vi "update.vi"(8 "error in (no error)":errorcluster, 10 "Model in":refnum<class "Model.lvclass">, 11 "DisabledState in":refnum<class "DisabledState.lvclass">) -> (0 "error out":errorcluster, 2 "Model out":refnum<class "Model.lvclass">, 3 "DisabledState out":refnum<class "DisabledState.lvclass">)   [LabVIEW 2016, in "DisabledState.lvclass"]
uses:
  DisabledState.lvclass
  Model/Model.lvclass
  Model/Model.lvclass/Model.ctl
  ILCCommunications/ILCCommunications.lvclass/ILCCommunications.ctl
  Common_RT_HPILC/HPILC/HPILC.lvclass/HPILC.ctl
  Common_RT_ILC/ILC/ILC.lvclass/ILC.ctl
  Common_RT_Modbus/ModbusBuffer/ModbusBuffer.lvclass/ModbusBuffer.ctl
  Common_RT_FAILC/FAILC/FAILC.lvclass/FAILC.ctl
  Publisher/Publisher.lvclass/Publisher.ctl
  Communicator/M1M3SAL/M1M3SAL.lvclass/M1M3SAL.ctl
  ILCCommunications/broadcastHPFreezeSensorValues.vi
  ILCCommunications/broadcastFAFreezeSensorValues.vi
  ILCCommunications/reportAllHPForceAndStatus.vi
  ILCCommunications/reportAllFAForceAndStatus.vi
  ILCCommunications/reportAllHPServerStatus.vi
  Model/getFPGA.vi
  Model/setFPGA.vi
  ILCCommunications/parse.vi
  Publisher/transmit.vi
  Common_RT_HPILC/HPILC/addBroadcastFreezeSensorValuesFrame.vi
  Common_RT_FAILC/FAILC/addBroadcastFreezeSensorValuesFrame.vi
  ILCCommunications/reportHPForceAndStatus.vi
  ILCCommunications/reportFAForceAndStatus.vi
  ILCCommunications/reportHPServerStatus.vi
  Common_RT_Modbus/ModbusBuffer/endOfBuffer.vi
  Common_RT_Modbus/ModbusBuffer/readHeader.vi
  Common_RT_Modbus/ModbusBuffer/readU8.vi
  ILCCommunications/findILCMap.vi
  ILCCommunications/getHPs.vi
  ILCCommunications/setHPs.vi
  Common_RT_HPILC/HPILC/parseHP.vi
  ILCCommunications/getFAs.vi
  ILCCommunications/setFAs.vi
  Common_RT_FAILC/FAILC/parseFA.vi
  Communicator/M1M3SAL/transmit.vi
  Common_RT_Modbus/ModbusBuffer/writeHeader.vi
  Common_RT_Modbus/ModbusBuffer/writeU8.vi
  Common_RT_Modbus/ModbusBuffer/writeCRC.vi
  Common_RT_Modbus/ModbusBuffer/writeDelay.vi
  Common_RT_ILC/ILC/getILCData.vi
  Common_RT_Modbus/ModbusBuffer/writeEndOfFrame.vi
  Common_RT_HPILC/HPILC/createForceAndStatusFrame.vi
  Common_RT_FAILC/FAILC/addForceAndStatusFrame.vi
  ILCCommunications/reportServerStatus.vi
  Common_RT_Modbus/ModbusBuffer/readInstructionByte.vi
  ILCCommunications/getILCMap.vi
  Common_RT_ILC/ILC/parseILC.vi
  Common_RT_HPILC/HPILC/parseStepMotorResponse.vi
  Common_RT_HPILC/HPILC/parseStepMotorError.vi
  Common_RT_HPILC/HPILC/parseForceAndStatusResponse.vi
  Common_RT_HPILC/HPILC/parseForceAndStatusError.vi
  Common_RT_FAILC/FAILC/parseBoosterValveGainResponse.vi
  Common_RT_FAILC/FAILC/parseBoosterValveGainError.vi
  Common_RT_FAILC/FAILC/parseReadBoosterValveGainResponse.vi
  Common_RT_FAILC/FAILC/parseReadBoosterValveGainError.vi
  Common_RT_FAILC/FAILC/parseSetForceResponse.vi
  Common_RT_FAILC/FAILC/parseSetForceError.vi
  Common_RT_FAILC/FAILC/parseForceAndStatusResponse.vi
  Common_RT_FAILC/FAILC/parseForceAndStatusError.vi
  Communicator/M1M3SAL/write.vi
  Common_RT_Modbus/ModbusBuffer/writeByteInstruction.vi
  Common_RT_Modbus/ModbusBuffer/calculateCRC.vi
  Common_RT_Modbus/ModbusBuffer/writeWaitForRx.vi
  Common_RT_ILC/ILC/addReportServerStatusFrame.vi
  Common_RT_ILC/ILC/parseReportServerIDFrame.vi
  Common_RT_ILC/ILC/parseReportServerIDError.vi
  Common_RT_ILC/ILC/parseReportServerStatusFrame.vi
  Common_RT_ILC/ILC/parseReportServerStatusError.vi
  Common_RT_ILC/ILC/parseModeFrame.vi
  Common_RT_ILC/ILC/parseModeError.vi
  Common_RT_ILC/ILC/parseTemporaryAddressFrame.vi
  Common_RT_ILC/ILC/parseTemporaryAddressError.vi
  Common_RT_ILC/ILC/parseADCScanRateFrame.vi
  Common_RT_ILC/ILC/parseADCScanRateError.vi
  Common_RT_ILC/ILC/parseADCOffsetSensitivityFrame.vi
  Common_RT_ILC/ILC/parseADCOffsetSensitivityError.vi
  Common_RT_ILC/ILC/parseResetFrame.vi
  Common_RT_ILC/ILC/parseResetError.vi
  Common_RT_ILC/ILC/parseReportCalibrationDataFrame.vi
  Common_RT_ILC/ILC/parseReportCalibrationDataError.vi
  Common_RT_Modbus/ModbusBuffer/readCRC.vi
  Common_RT_Modbus/ModbusBuffer/readTimestamp.vi
  Common_RT_Modbus/ModbusBuffer/readEndOfFrame.vi
  Common_RT_Modbus/ModbusBuffer/readI32.vi
  Common_RT_Modbus/ModbusBuffer/readSGL.vi
  Common_RT_Modbus/ModbusBuffer/readU48.vi
  Common_RT_Modbus/ModbusBuffer/readString.vi
  Common_RT_Modbus/ModbusBuffer/readU16.vi
  Common_RT_Modbus/ModbusBuffer/readTimestampByte.vi
  Common_RT_HPILC/HPILC/HPILC.lvclass
  D:/Code/ts_M1M3Support/Common_RT_ILC/ILC/ILC.lvclass
  Common_RT_FAILC/FAILC/FAILC.lvclass
  Resources/FPGA/writeModbusTxData.vi
  Resources/FPGA/writeModbusTrigger.vi
  Resources/FPGA/writeHealthAndStatusControl.vi
  Resources/FPGA/readModbusRxData.vi
panel:
  out "Total Time (us)":u32
  out "Times (us)":u32[](array[numeric])
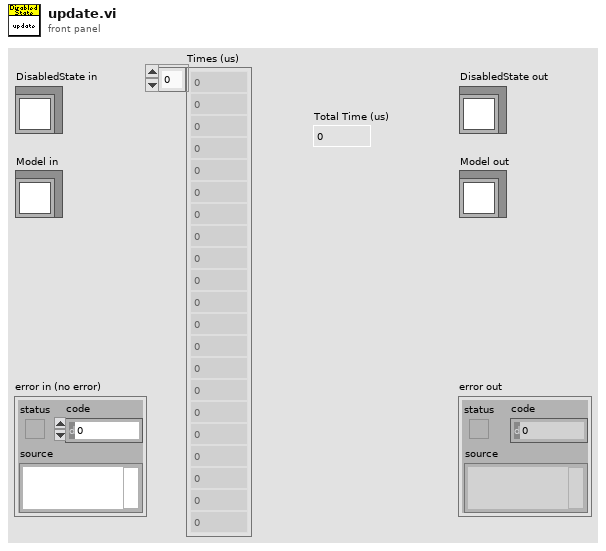
[diagram p1: front panel]
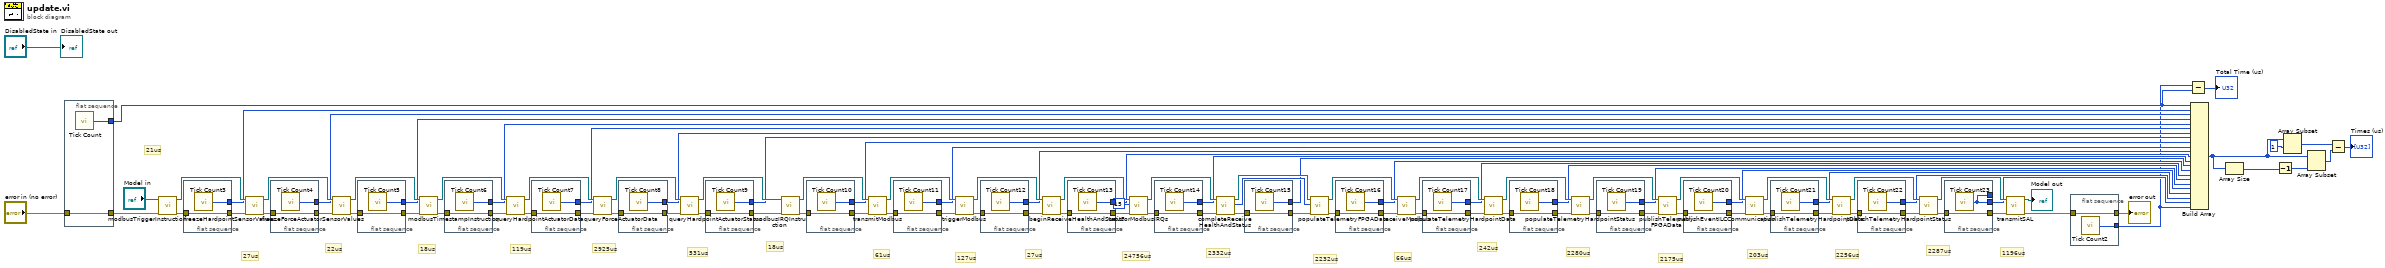
[diagram p0: block diagram]
diagram:
  # "1196us"
  # "2287us"
  # "2256us"
  # "203us"
  # "2175us"
  # "2280us"
  # "242us"
  # "66us"
  # "2232us"
  # "2332us"
  # "24756us"
  # "27us"
  # "127us"
  # "61us"
  # "531us"
  # "2925us"
  # "119us"
  # "18us"
  # "22us"
  # "27us"
  # "21us"
  # "18us"
  n1 = flat-sequence {
    tunnel: "error in (no error)" -> [w104]
    tunnel: [w105] -> w4
    tunnel: [w104] -> w79
    frame #0 {
      n2 = call "Tick Count"() -> ("Tick Count(uSec)"=w105:u32)
    }
  }
  n3 = call "modbusTriggerInstruction.vi"("error in (no error)"=w79, "Model in"="Model in") -> ("error out"=w75:errorcluster, "Model out"=w90:refnum<class "Model.lvclass">)  [unwired: 8 in]
  n4 = flat-sequence {
    tunnel: w75 -> [w107]
    tunnel: [w106] -> w67
    tunnel: [w107] -> w74
    frame #0 {
      n5 = call "Tick Count3"() -> ("Tick Count(uSec)"=w106:u32)
    }
  }
  n6 = call "freezeHardpointSensorValues.vi"("error in (no error)"=w74, "Model in"=w90) -> ("error out"=w73:errorcluster, "Model out"=w84:refnum<class "Model.lvclass">)  [unwired: 8 in]
  n7 = flat-sequence {
    tunnel: w73 -> [w109]
    tunnel: [w108] -> w66
    tunnel: [w109] -> w72
    frame #0 {
      n8 = call "Tick Count4"() -> ("Tick Count(uSec)"=w108:u32)
    }
  }
  n9 = call "freezeForceActuatorSensorValues.vi"("error in (no error)"=w72, "Model in"=w84) -> ("error out"=w71:errorcluster, "Model out"=w83:refnum<class "Model.lvclass">)  [unwired: 8 in]
  n10 = flat-sequence {
    tunnel: w71 -> [w111]
    tunnel: [w110] -> w65
    tunnel: [w111] -> w70
    frame #0 {
      n11 = call "Tick Count5"() -> ("Tick Count(uSec)"=w110:u32)
    }
  }
  n12 = call "modbusTimestampInstruction.vi"("error in (no error)"=w70, "Model in"=w83) -> ("error out"=w69:errorcluster, "Model out"=w91:refnum<class "Model.lvclass">)  [unwired: 8 in]
  n13 = flat-sequence {
    tunnel: w69 -> [w113]
    tunnel: [w112] -> w64
    tunnel: [w113] -> w68
    frame #0 {
      n14 = call "Tick Count6"() -> ("Tick Count(uSec)"=w112:u32)
    }
  }
  n15 = call "queryHardpointActuatorData.vi"("error in (no error)"=w68, "Model in"=w91) -> ("error out"=w63:errorcluster, "Model out"=w82:refnum<class "Model.lvclass">)  [unwired: 8 in]
  n16 = flat-sequence {
    tunnel: w63 -> [w115]
    tunnel: [w114] -> w57
    tunnel: [w115] -> w62
    frame #0 {
      n17 = call "Tick Count7"() -> ("Tick Count(uSec)"=w114:u32)
    }
  }
  n18 = call "queryForceActuatorData.vi"("error in (no error)"=w62, "Model in"=w82) -> ("error out"=w61:errorcluster, "Model out"=w81:refnum<class "Model.lvclass">)  [unwired: 8 in]
  n19 = flat-sequence {
    tunnel: w61 -> [w117]
    tunnel: [w116] -> w56
    tunnel: [w117] -> w60
    frame #0 {
      n20 = call "Tick Count8"() -> ("Tick Count(uSec)"=w116:u32)
    }
  }
  n21 = call "queryHardpointActuatorStatus.vi"("error in (no error)"=w60, "Model in"=w81) -> ("error out"=w59:errorcluster, "Model out"=w94:refnum<class "Model.lvclass">)  [unwired: 8 in]
  n22 = flat-sequence {
    tunnel: w59 -> [w119]
    tunnel: [w118] -> w55
    tunnel: [w119] -> w58
    frame #0 {
      n23 = call "Tick Count9"() -> ("Tick Count(uSec)"=w118:u32)
    }
  }
  n24 = call "modbusIRQInstruction.vi"("error in (no error)"=w58, "Model in"=w94) -> ("error out"=w54:errorcluster, "Model out"=w93:refnum<class "Model.lvclass">)  [unwired: 8 in]
  n25 = flat-sequence {
    tunnel: w54 -> [w121]
    tunnel: [w120] -> w40
    tunnel: [w121] -> w53
    frame #0 {
      n26 = call "Tick Count10"() -> ("Tick Count(uSec)"=w120:u32)
    }
  }
  n27 = call "transmitModbus.vi"("error in (no error)"=w53, "Model in"=w93) -> ("error out"=w52:errorcluster, "Model out"=w92:refnum<class "Model.lvclass">)  [unwired: 8 in]
  n28 = flat-sequence {
    tunnel: w52 -> [w123]
    tunnel: [w122] -> w39
    tunnel: [w123] -> w51
    frame #0 {
      n29 = call "Tick Count11"() -> ("Tick Count(uSec)"=w122:u32)
    }
  }
  n30 = call "triggerModbus.vi"("error in (no error)"=w51, "Model in"=w92) -> ("error out"=w50:errorcluster, "Model out"=w89:refnum<class "Model.lvclass">)  [unwired: 8 in]
  n31 = flat-sequence {
    tunnel: w50 -> [w125]
    tunnel: [w124] -> w38
    tunnel: [w125] -> w49
    frame #0 {
      n32 = call "Tick Count12"() -> ("Tick Count(uSec)"=w124:u32)
    }
  }
  n33 = call "beginReceiveHealthAndStatus.vi"("error in (no error)"=w49, "Model in"=w89) -> ("error out"=w48:errorcluster, "Model out"=w102:refnum<class "Model.lvclass">)  [unwired: 8 in]
  n34 = flat-sequence {
    tunnel: w48 -> [w127]
    tunnel: [w126] -> w37
    tunnel: [w127] -> w47
    frame #0 {
      n35 = call "Tick Count13"() -> ("Tick Count(uSec)"=w126:u32)
    }
  }
  n36 = call "waitForModbusIRQs.vi"("error in (no error)"=w47, "Timeout (ms)"=15, "Model in"=w102) -> ("error out"=w46:errorcluster, "Model out"=w88:refnum<class "Model.lvclass">)  [unwired: 7 in]
  n37 = flat-sequence {
    tunnel: w46 -> [w129]
    tunnel: [w128] -> w36
    tunnel: [w129] -> w45
    frame #0 {
      n38 = call "Tick Count14"() -> ("Tick Count(uSec)"=w128:u32)
    }
  }
  n39 = call "completeReceiveHealthAndStatus.vi"("error in (no error)"=w45, "Model in"=w88) -> ("error out"=w44:errorcluster, "Data"=w101:u64[], "Model out"=w100:refnum<class "Model.lvclass">)  [unwired: 7 in]
  n40 = flat-sequence {
    tunnel: w44 -> [w131]
    tunnel: [w130] -> w35
    tunnel: [w131] -> w43
    frame #0 {
      n41 = call "Tick Count15"() -> ("Tick Count(uSec)"=w130:u32)
    }
  }
  n42 = call "populateTelemetryFPGAData.vi"("error in (no error)"=w43, "Data"=w101, "Model in"=w100) -> ("error out"=w42:errorcluster, "Model out"=w87:refnum<class "Model.lvclass">)  [unwired: 7 in]
  n43 = flat-sequence {
    tunnel: w42 -> [w133]
    tunnel: [w132] -> w34
    tunnel: [w133] -> w41
    frame #0 {
      n44 = call "Tick Count16"() -> ("Tick Count(uSec)"=w132:u32)
    }
  }
  n45 = call "receiveModbus.vi"("error in (no error)"=w41, "Model in"=w87) -> ("error out"=w33:errorcluster, "Model out"=w86:refnum<class "Model.lvclass">)  [unwired: 8 in]
  n46 = flat-sequence {
    tunnel: w33 -> [w135]
    tunnel: [w134] -> w18
    tunnel: [w135] -> w32
    frame #0 {
      n47 = call "Tick Count17"() -> ("Tick Count(uSec)"=w134:u32)
    }
  }
  n48 = call "populateTelemetryHardpointData.vi"("error in (no error)"=w32, "Model in"=w86) -> ("error out"=w31:errorcluster, "Model out"=w99:refnum<class "Model.lvclass">)  [unwired: 8 in]
  n49 = flat-sequence {
    tunnel: w31 -> [w137]
    tunnel: [w136] -> w17
    tunnel: [w137] -> w30
    frame #0 {
      n50 = call "Tick Count18"() -> ("Tick Count(uSec)"=w136:u32)
    }
  }
  n51 = call "populateTelemetryHardpointStatus.vi"("error in (no error)"=w30, "Model in"=w99) -> ("error out"=w29:errorcluster, "Model out"=w97:refnum<class "Model.lvclass">)  [unwired: 8 in]
  n52 = flat-sequence {
    tunnel: w29 -> [w139]
    tunnel: [w138] -> w16
    tunnel: [w139] -> w28
    frame #0 {
      n53 = call "Tick Count19"() -> ("Tick Count(uSec)"=w138:u32)
    }
  }
  n54 = call "publishTelemetryFPGAData.vi"("error in (no error)"=w28, "Model in"=w97) -> ("error out"=w27:errorcluster, "Model out"=w96:refnum<class "Model.lvclass">)  [unwired: 8 in]
  n55 = flat-sequence {
    tunnel: w27 -> [w141]
    tunnel: [w140] -> w15
    tunnel: [w141] -> w26
    frame #0 {
      n56 = call "Tick Count20"() -> ("Tick Count(uSec)"=w140:u32)
    }
  }
  n57 = call "publishEventILCCommunication.vi"("error in (no error)"=w26, "Model in"=w96) -> ("error out"=w25:errorcluster, "Model out"=w95:refnum<class "Model.lvclass">)  [unwired: 8 in]
  n58 = flat-sequence {
    tunnel: w25 -> [w143]
    tunnel: [w142] -> w14
    tunnel: [w143] -> w24
    frame #0 {
      n59 = call "Tick Count21"() -> ("Tick Count(uSec)"=w142:u32)
    }
  }
  n60 = call "publishTelemetryHardpointData.vi"("error in (no error)"=w24, "Model in"=w95) -> ("error out"=w23:errorcluster, "Model out"=w98:refnum<class "Model.lvclass">)  [unwired: 8 in]
  n61 = flat-sequence {
    tunnel: w23 -> [w145]
    tunnel: [w144] -> w13
    tunnel: [w145] -> w22
    frame #0 {
      n62 = call "Tick Count22"() -> ("Tick Count(uSec)"=w144:u32)
    }
  }
  n63 = call "publishTelemetryHardpointStatus.vi"("error in (no error)"=w22, "Model in"=w98) -> ("error out"=w21:errorcluster, "Model out"=w77:refnum<class "Model.lvclass">)  [unwired: 8 in]
  n64 = flat-sequence {
    tunnel: w21 -> [w147]
    tunnel: [w146] -> _
    tunnel: [w147] -> w20
    tunnel: [w146] -> w12
    frame #0 {
      n65 = call "Tick Count23"() -> ("Tick Count(uSec)"=w146:u32)
    }
  }
  n66 = call "transmitSAL.vi"("error in (no error)"=w20, "Model in"=w77) -> ("error out"=w78:errorcluster, "Model out"=→"Model out":refnum<class "Model.lvclass">)  [unwired: 8 in]
  n67 = flat-sequence {
    tunnel: w78 -> [w148]
    tunnel: [w149] -> w3
    tunnel: [w148] -> w19
    frame #0 {
      n68 = call "Tick Count2"() -> ("Tick Count(uSec)"=w149:u32)
    }
  }
  n69 = Subtract(x=w3, y=w4) -> (x-y=→"Total Time (us)":u32)
  n70 = Build Array(w4, w67, w66, w65, w64, w57, w56, w55, w40, w39, w38, w37, w36, w35, w34, w18, w17, w16, w15, w14, w13, w12, w3) -> (w11:u32[])
  n71 = Array Size(array=w11) -> (size(s)=w10:i32)
  n72 = Decrement(x=w10) -> (x-1=w9:i32)
  n73 = Array Subset(array=w11, index=1) -> (w7:u32[])  [unwired: 1 in]
  n74 = Array Subset(array=w11, length=w9) -> (w6:u32[])  [unwired: 1 in]
  n75 = Subtract(x=w7, y=w6) -> (x-y=→"Times (us)":u32[])
  "error out" <- w19
  "DisabledState out" <- "DisabledState in"
